vi "FT_Read_String_Data.vi"(8 "error in":errorcluster, 10 "Bytes To Read":u32, 11 "Handle":u32) -> (0 "error out":errorcluster, 1 "Bytes Read":u32, 2 "Read Data":string, 3 "Handle out":u32)   [LabVIEW 2016]
uses:
  FTD2XX.dll
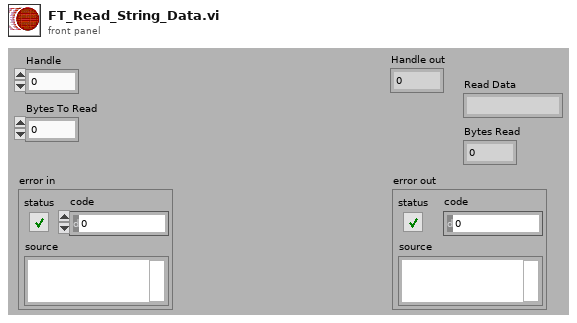
[diagram p1: front panel]
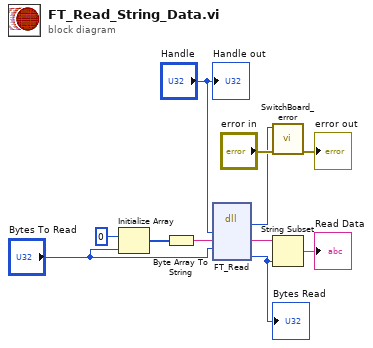
[diagram p0: block diagram]
diagram:
  n1 = Initialize Array(u8 0, "Bytes To Read") -> (w10:u8[])
  n2 = Byte Array To String(unsigned byte array=w10) -> (string=w9:string)
  n3 = dll-call lib="FTD2XX.dll" fn="FT_Read"("Handle"="Handle", "Buffer"=w9, "BytesToRead"="Bytes To Read") -> ("FT_Status"=w1:u32, "Buffer"=w6:string, "BytesReturned"=w5:u32)  [unwired: 6 in, 2 out]
  "Bytes Read" <- w5
  n4 = call <instrlib>:"SwitchBoard_error.vi"("error constant"="error in", "Code"=w1) -> ("error IO"=→"error out":errorcluster)  [unwired: 9 in]
  n5 = String Subset(string=w6, length (rest)=w5) -> (substring=→"Read Data":string)  [unwired: 1 in]
  "Handle out" <- "Handle"
